vi "Live view.vi"(7 "Timings Array":u64[](array[numeric]), 8 "error in (no error)":errorcluster, 10 "dst image":T2, 11 "CamSession in":T1) -> (0 "error out":errorcluster, 1 "Frame Rate (Hz)":dbl, 2 "Image out":T2, 3 "CamSession Out":T1, 4 "Image Saturated":bool, 5 "Timings Array out":u64[](array[numeric]), 6 "ImgHist":u32[](graph))   [LabVIEW 2020]
uses:
  <vilib>/vision/Image Controls.llb/IMAQ Image.ctl
  <vilib>/userDefined/High Color/IMAQdx.ctl
  _controls/Timer_actions.ctl
  <vilib>/vision/driver/NI_Vision_Acquisition_Software.lvlib
panel:
  in  "Draw Spots":bool=TRUE
  in  "MicronsPerPx":dbl=0.277 format="%#_13g"
  in  "Spot Radius":dbl=3.0 format="%#_13g"
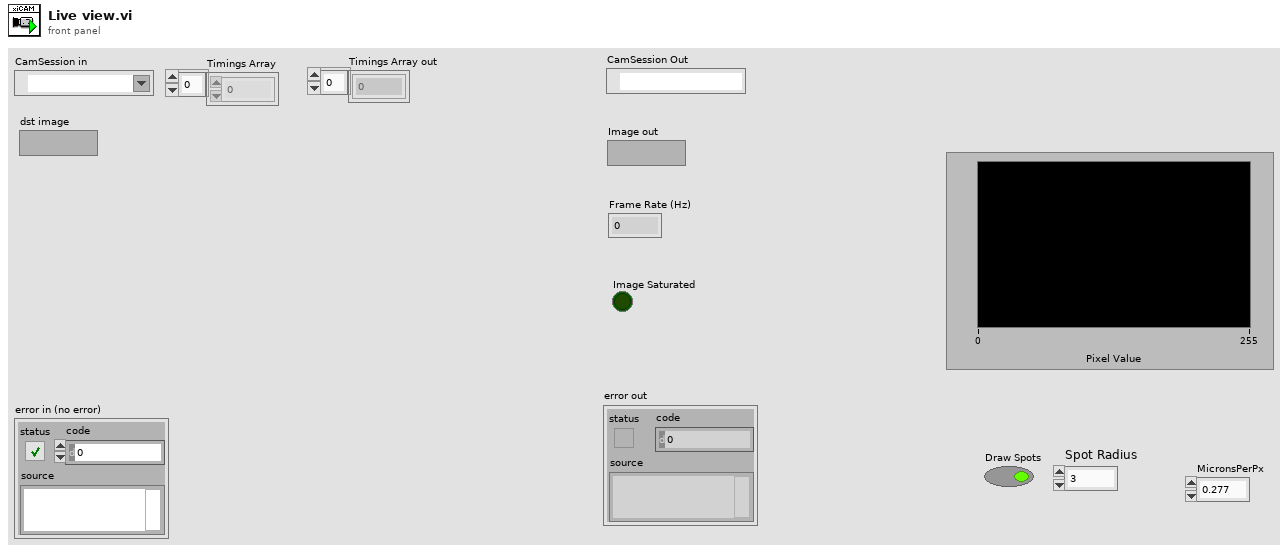
[diagram p1: front panel]
types:
  T1 = typedef "IMAQdx.ctl" = refnum<k21>
  T2 = typedef "IMAQ Image.ctl" = refnum<image>
  T3 = typedef "Timer_actions.ctl" = enum16{"Reset", "Snap", "Total"}
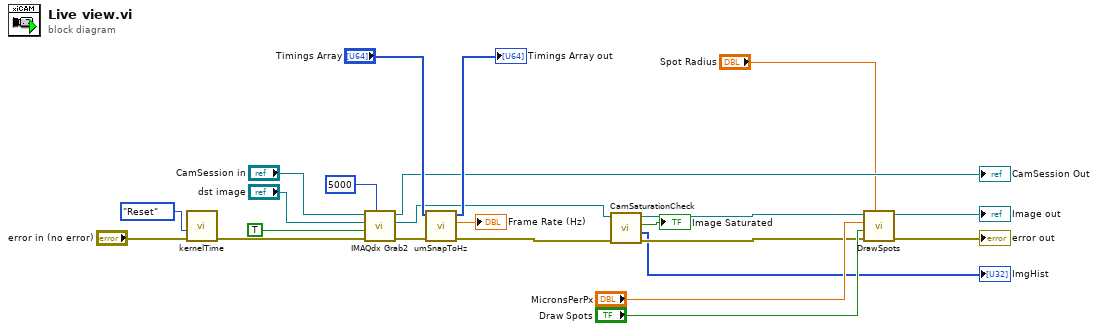
[diagram p0: block diagram]
diagram:
  n1 = call "kernelTime.vi"("error in (no error) in"="error in (no error)", "Action (Snap)"=Timer_actions."Reset") -> ("error out"=w7:errorcluster)  [unwired: 8 in, 1 out]
  n2 = call <vilib>:"IMAQdx Grab2.vi"("Timeout (ms)"=5000, "error in"=w7, "Wait for Next Buffer? (Yes)"=TRUE, "Image In"="dst image", "Session In"="CamSession in") -> ("error out"=w6:errorcluster, "Image Out"=w16:T2, "Session Out"=→"CamSession Out":T1)  [unwired: 3 in, 1 out]
  n3 = call "umSnapToHz.vi"("error in (no error)"=w6, "Snap Buffer (um) in"="Timings Array") -> ("error out"=w5:errorcluster, "Frame Rate (Hz)"=→"Frame Rate (Hz)":dbl, "Snap Buffer(um) out"=→"Timings Array out":u64[])  [unwired: 7 in]
  n4 = call "CamSaturationCheck.vi"("error in (no error)"=w5, "Img In"=w16) -> ("error out"=w4:errorcluster, "ImgHist"=→"ImgHist":u32[], "Image Saturated"=→"Image Saturated":bool, "Img out"=w15:T2)  [unwired: 6 in]
  n5 = call "DrawSpots.vi"("Spot Radius"="Spot Radius", "error in (no error)"=w4, "Draw Spots"="Draw Spots", "MicronsPerPx"="MicronsPerPx", "img in"=w15) -> ("error out"=→"error out":errorcluster, "img out"=→"Image out":T2)  [unwired: 5 in]
